vi "Core Actor - CLOSE  - ALL Control References.vi"(8 "error in (no error)":errorcluster, 11 "Child_2_Class in":refnum<class "SW_Interface_Class.lvclass">) -> (0 "error out":errorcluster, 3 "Child_2_Class out":refnum<class "SW_Interface_Class.lvclass">)   [LabVIEW 2023, in "SW_Interface_Actor.lvlib" / "SW_Interface_Class.lvclass"]
uses:
  SW_Interface_Class.lvclass
  SW_Interface_Class.lvclass/SW_Interface_Class.ctl
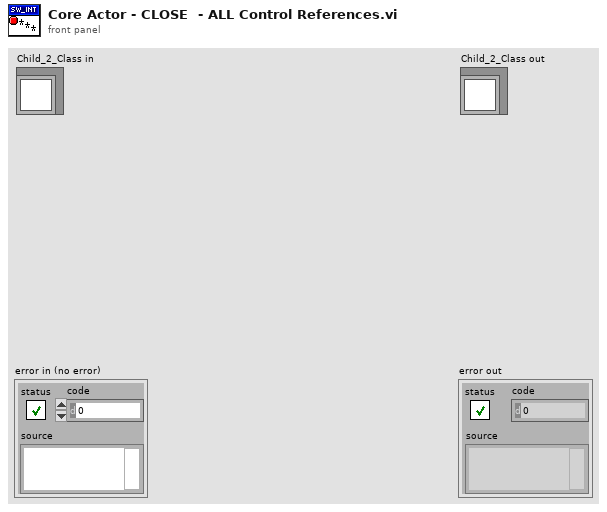
[diagram p1: front panel]
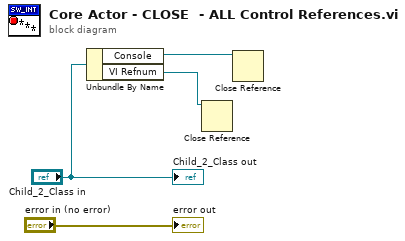
[diagram p0: block diagram]
diagram:
  n1 = Unbundle By Name("Child_2_Class in") -> ("Console"=w3:refnum<vi>, "VI Refnum"=w2:refnum<vi>)
  n2 = Close Reference(reference=w2) -> ()  [unwired: 1 in, 1 out]
  n3 = Close Reference(reference=w3) -> ()  [unwired: 1 in, 1 out]
  "error out" <- "error in (no error)"
  "Child_2_Class out" <- "Child_2_Class in"
